vi "LinearSystemId_DCMotor_Pack_Model_Params.vi"(5 "DCMOTOR_TYPES":T2, 7 "Num Motors":i32=1, 10 "MOI kgm2":dbl=0.0001, 11 "Gearing":dbl=1.0) -> (3 "LinearSystem_ID_DCMotor_Model":T1 {"MOI kgm2" format="%#_13g"; "Gearing" format="%#_13g"})   [LabVIEW 2019, in "Trajectory_Library.lvlib"]
uses:
  Trajectory_Library.lvlib
  Enum/DCMOTOR_TYPES_ENUM.ctl
  TypeDef/LINEAR_SYSTEM_ID_DCMOTOR_MODEL.ctl
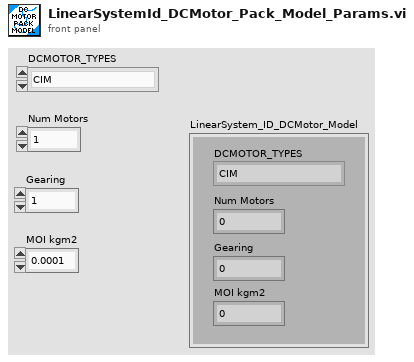
[diagram p1: front panel]
types:
  T1 = typedef "Trajectory_Library.lvlib/LINEAR_SYSTEM_ID_DCMOTOR_MODEL.ctl" = cluster{"DCMOTOR_TYPES":T2, "Num Motors":i32, "Gearing":dbl, "MOI kgm2":dbl}
  T2 = typedef "Trajectory_Library.lvlib/DCMOTOR_TYPES_ENUM.ctl" = enum16{"CIM", "AndyMark 9015", "Andy Mark RS 775 125", "Bag", "BaneBots RS 550", "BaneBots RS 775", "Falcon 500", "Mini CIM", "NEO", "NEO 550", "Romi BuiltIn", "Vex 775 Pro", "Snow Blower AM 2235A", "Bosch Seat AM 3493"}
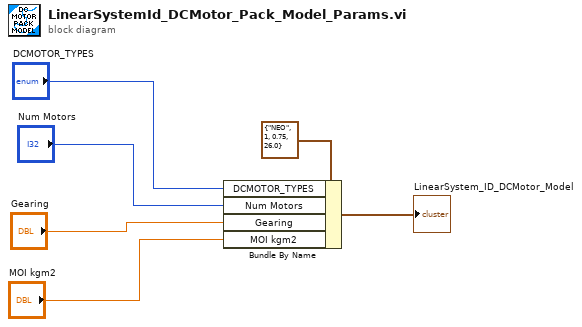
[diagram p0: block diagram]
diagram:
  n1 = Bundle By Name(cluster=T1 {"DCMOTOR_TYPES"=enum."NEO", "Num Motors"=1, "Gearing"=0.75, "MOI kgm2"=26.0} ("DCMotorSim_Model _Params"), "DCMOTOR_TYPES"="DCMOTOR_TYPES", "Num Motors"="Num Motors", "Gearing"="Gearing", "MOI kgm2"="MOI kgm2") -> (→"LinearSystem_ID_DCMotor_Model":T1)
